vi "RebootLogName.vi"() -> (1 "reboot log name":string)   [LabVIEW 2017, in "Controller.lvlib"]
uses:
  <vilib>/addons/InsightCM/Devices/Shared/Common/Controller/Controller.lvlib
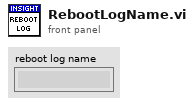
[diagram p1: front panel]
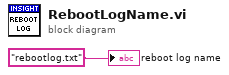
[diagram p0: block diagram]
diagram:
  "reboot log name" <- "rebootlog.txt" ("name or relative path")
